vi "Save Buffered Data.vi"(8 "error in (no error)":errorcluster, 11 "Calling Actor in":refnum<class "Calling Actor.lvclass">) -> (0 "error out":errorcluster, 3 "Calling Actor out":refnum<class "Calling Actor.lvclass">)   [LabVIEW 2020, in "Calling Actor.lvlib" / "Calling Actor.lvclass"]
uses:
  Calling Actor.lvclass
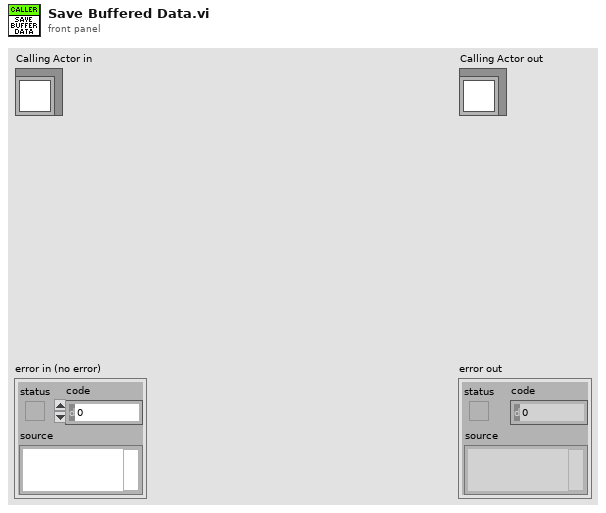
[diagram p1: front panel]
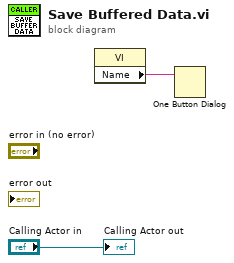
[diagram p0: block diagram]
diagram:
  n1 = property class="VI"() -> ("Name"=w1:string)  [unwired: 2 in, 2 out]
  n2 = One Button Dialog(message=w1) -> ()  [unwired: 1 in, 1 out]
  "Calling Actor out" <- "Calling Actor in"
